vi "Create.vi"(7 "VolatusAPI":refnum<class "VolatusAPI.lvclass">, 8 "error in (no error)":errorcluster, 10 "Channel":string) -> (0 "error out":errorcluster, 3 "Numeric Command out":refnum<class "Numeric Command.lvclass">)   [LabVIEW 2020, in "Volatus.lvlib" / "Numeric Command.lvclass"]
uses:
  Numeric Command.lvclass
  Numeric Command.lvclass/Numeric Command.ctl
  VolatusAPI/VolatusAPI.lvclass
  messages/CmdAnalog/Data.ctl
  messages/CmdAnalog/CmdAnalog.lvlib
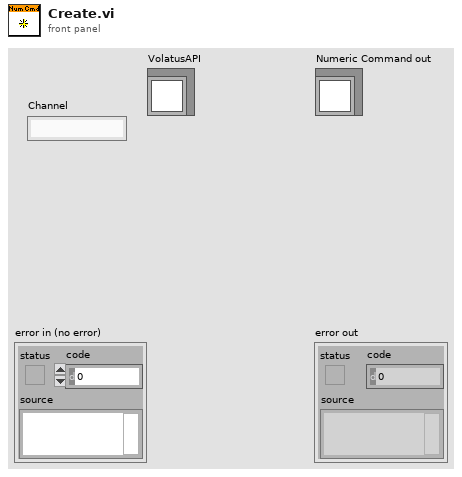
[diagram p1: front panel]
types:
  T1 = typedef "CmdAnalog.lvlib/Data.ctl" = cluster{"channel":string, "value":dbl}
  T2 = typedef "VectoConfig.lvlib/Channel Info.ctl" = cluster{"Name":string, "Group":string, "Owning Node":string, "Owning Task":string, "Resource":string}
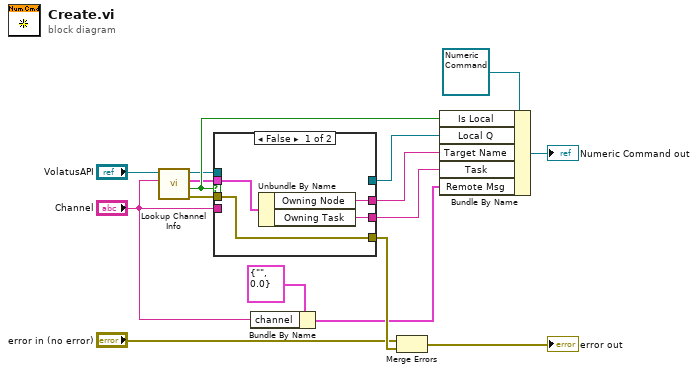
[diagram p0: block diagram]
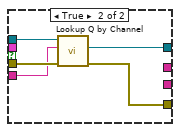
[diagram p2: hidden frame]
diagram:
  n1 = call "Lookup Channel Info.vi"("Channel Name"="Channel", "VolatusAPI in"="VolatusAPI") -> ("error out"=w5:errorcluster, "Local"=w14:bool, "Channel Info"=w8:T2, "VolatusAPI out"=w13:refnum<class "VolatusAPI.lvclass">)  [unwired: 6 in]
  n2 = case shown="False" w14 {
    tunnel: w13 -> [_ w24]
    tunnel: "Channel" -> [_ w23]
    tunnel: [_ w22] -> w11
    tunnel: w8 -> [w20 _]
    tunnel: [w19 _] -> w7
    tunnel: [w18 _] -> w6
    tunnel: w5 -> [w17 w25]
    tunnel: [w17 w21] -> w16
    frame False {
      n3 = Unbundle By Name(w20) -> ("Owning Node"=w19:string, "Owning Task"=w18:string)
    }
    frame True {
      n4 = call "Lookup Q by Channel.vi"("error in (no error)"=w25, "Channel Name"=w23, "VolatusAPI in"=w24) -> ("error out"=w21:errorcluster, "MessageQ"=w22:refnum<class "MessageQ.lvclass">)  [unwired: 6 in, 1 out]
    }
  }
  n5 = Bundle By Name(cluster=T1 {"channel"="", "value"=0.0} ("Remote Msg"), "channel"="Channel") -> (w9:T1)
  n6 = Merge Errors("error in (no error)", w16) -> (→"error out":errorcluster)
  n7 = Bundle By Name(cluster=refnum<class "Numeric Command.lvclass"> refnum ("Numeric Command in"), "Is Local"=w14, "Local Q"=w11, "Target Name"=w7, "Task"=w6, "Remote Msg"=w9) -> (→"Numeric Command out":refnum<class "Numeric Command.lvclass">)
